vi "ICM aI8.vi"(11 "String In":string) -> (1 "Value I8":i8, 2 "Value":dbl, 3 "String Out":string)   [LabVIEW 2018]
doc: "OSDS aI8.vi\n\n This VI is used to parse binary data that contains a I8 integer.\n\nThis VI was original part of the OSDS system.\n\nInstrument Communication Module Version 1.0\nSeptember, 2017 Original Code Consulting David Thomson\n www.originalcode.com\n\n\nOSDS is licensed under the Creative Commons Attribution-Share Alike 3.0 license (http://creativecommons.org/). Derivative and commercial works incorporating OSDS are allowed, as long as changes you make are made available to the community at large. Please submit improvements as well as new OSDS Format Files and OSDS Stream Files to support@originalcode.com"
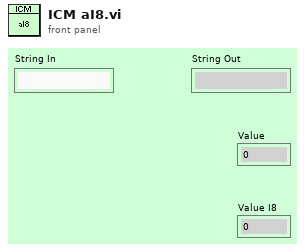
[diagram p1: front panel]
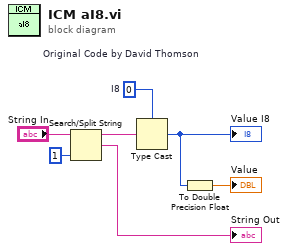
[diagram p0: block diagram]
diagram:
  w5 = i8 0  # I8
  n1 = Search/Split String(string="String In", offset (0)=1) -> (substring before match=w1:string, match + rest of string=→"String Out":string)  [unwired: 2 out]
  n2 = Type Cast "Original Code by David Thomson"(type=w5, x=w1) -> (*(type *) &x=w3:i8)
  "Value I8" <- w3
  n3 = To Double Precision Float(number=w3) -> (double precision float=→"Value":dbl)
